vi "OP Scaner Config.vi"(8 "error in (no error)":errorcluster, 9 "Enum":enum16{"init", "Read", "Write"}(ring)=enum."Read", 10 "VISA in":T1={"VISA"="", "baud rate"=9600, "data bits"=8, "parity"=enum."None", "stop bits"=10, "flow control"=0} {"flow control" items=["None", "XON/XOFF", "RTS/CTS", "XON/XOFF & RTS/CTS", "DTR/DSR", "XON/XOFF & DTR/DSR"]; "stop bits" items=["1.0"=10, "1.5"=15, "2.0"=20]}, 11 "Path":path) -> (0 "error out":errorcluster, 2 "VISA":T1={"VISA"="", "baud rate"=9600, "data bits"=8, "parity"=enum."None", "stop bits"=10, "flow control"=0} {"flow control" items=["None", "XON/XOFF", "RTS/CTS", "XON/XOFF & RTS/CTS", "DTR/DSR", "XON/XOFF & DTR/DSR"]; "stop bits" items=["1.0"=10, "1.5"=15, "2.0"=20]}, 3 "Path out":path)   [LabVIEW 2014]
uses:
  VISA/Ctr/VISA Ctr.ctl
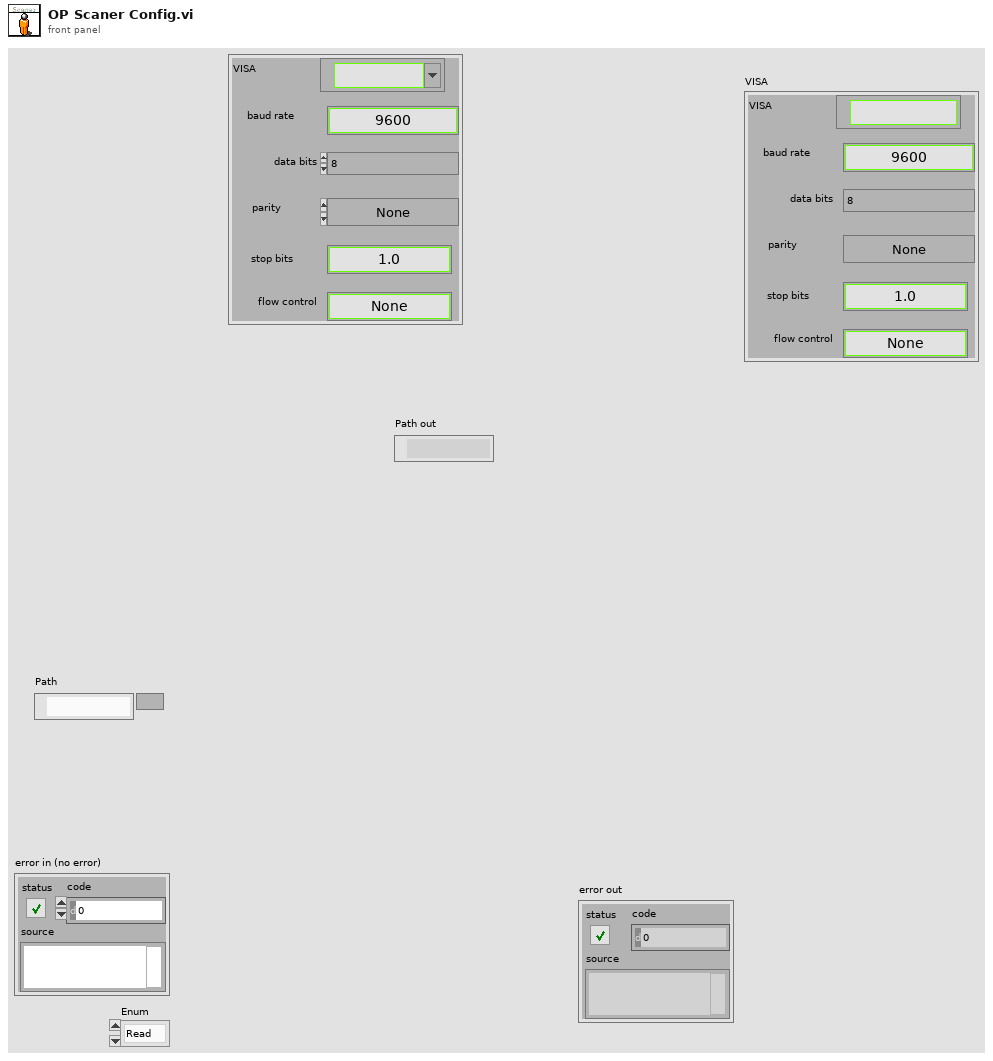
[diagram p1: front panel]
types:
  T1 = typedef "VISA Ctr.ctl" = cluster{"VISA":refnum<visa-resource-name>, "baud rate":u32, "data bits":u16, "parity":enum16{"None", "Odd", "Even", "Mark", "Space"}, "stop bits":u16, "flow control":u16}
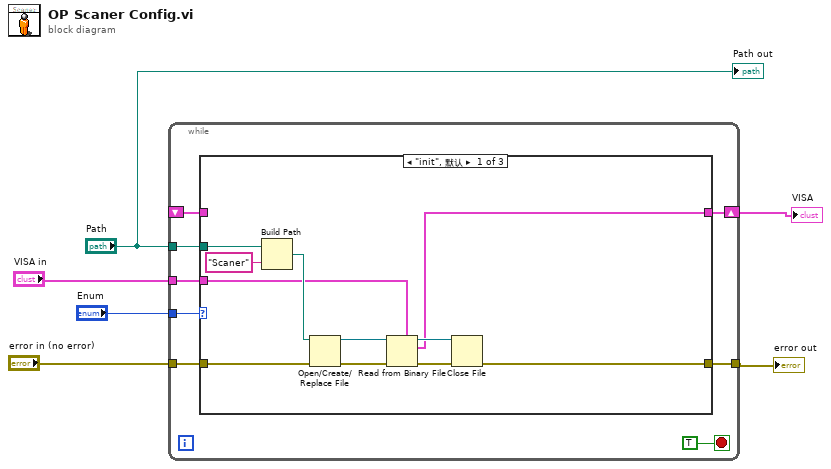
[diagram p0: block diagram]
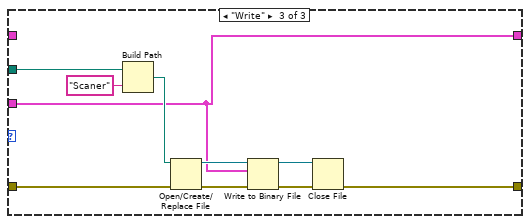
[diagram p3: hidden frame]
diagram:
  n1 = while {
    tunnel: "Enum" -> [w14]
    tunnel: "Path" -> [w13]
    tunnel: "error in (no error)" -> [w12]
    tunnel: "VISA in" -> [w11]
    shift-right: [w10] -> w1
    shift-left: _ -> [w8]
    tunnel: [w9] -> w3
    stop <- TRUE stop-if-true
    n2 = case shown="\"init\", 默认" w14 {
      tunnel: w13 -> [w24 _ w29]
      tunnel: w12 -> [w19 w26 w31]
      tunnel: w11 -> [w17 _ w28]
      tunnel: [w16 w27 w28] -> w10
      tunnel: [w15 w26 w30] -> w9
      tunnel: w8 -> [_ w27 _]
      frame "init", Default {
        n3 = Build Path(base path=w24, name or relative path="Scaner") -> (appended path=w18:path)
        n4 = Open/Create/Replace File(file path (use dialog)=w18, error in=w19) -> (refnum out=w23:refnum<file>, error out=w22:errorcluster)  [unwired: 4 in, 1 out]
        n5 = Read from Binary File(5:w17, 8:w22, 11:w23) -> (0:w20:errorcluster, 2:w16:T1, 3:w21:refnum<file>)  [unwired: 3 in, 1 out]
        n6 = Close File(refnum=w21, error in=w20) -> (error out=w15:errorcluster)  [unwired: 1 out]
      }
      frame "Read" {
      }
      frame "Write" {
        n7 = Build Path(base path=w29, name or relative path="Scaner") -> (appended path=w32:path)
        n8 = Open/Create/Replace File(file path (use dialog)=w32, error in=w31) -> (refnum out=w36:refnum<file>, error out=w35:errorcluster)  [unwired: 4 in, 1 out]
        n9 = Write to Binary File(file (use dialog)=w36, data=w28, error in=w35) -> (refnum out=w34:refnum<file>, error out=w33:errorcluster)  [unwired: 3 in, 1 out]
        n10 = Close File(refnum=w34, error in=w33) -> (error out=w30:errorcluster)  [unwired: 1 out]
      }
    }
  }
  "VISA" <- w1
  "error out" <- w3
  "Path out" <- "Path"
